vi "Configure Dialog.vi"(8 "error in (no error)":errorcluster, 11 "Get Auto Range Value [ARV] Msg.lvclass":refnum<class "Get Auto Range Value [ARV] Msg.lvclass">) -> (0 "error out":errorcluster, 2 "Ok?":bool, 3 "Get Auto Range Value [ARV] Msg.lvclass":refnum<class "Get Auto Range Value [ARV] Msg.lvclass">)   [LabVIEW 2015, in "CS++DMM.lvlib" / "Get Auto Range Value [ARV] Msg.lvclass"]
uses:
  Get Auto Range Value [ARV] Msg.lvclass
  Get Auto Range Value [ARV] Msg.lvclass/Get Auto Range Value [ARV] Msg.ctl
panel:
  in  "Execute?":bool
  in  "Cancel Button":bool
  in  "OK Button":bool
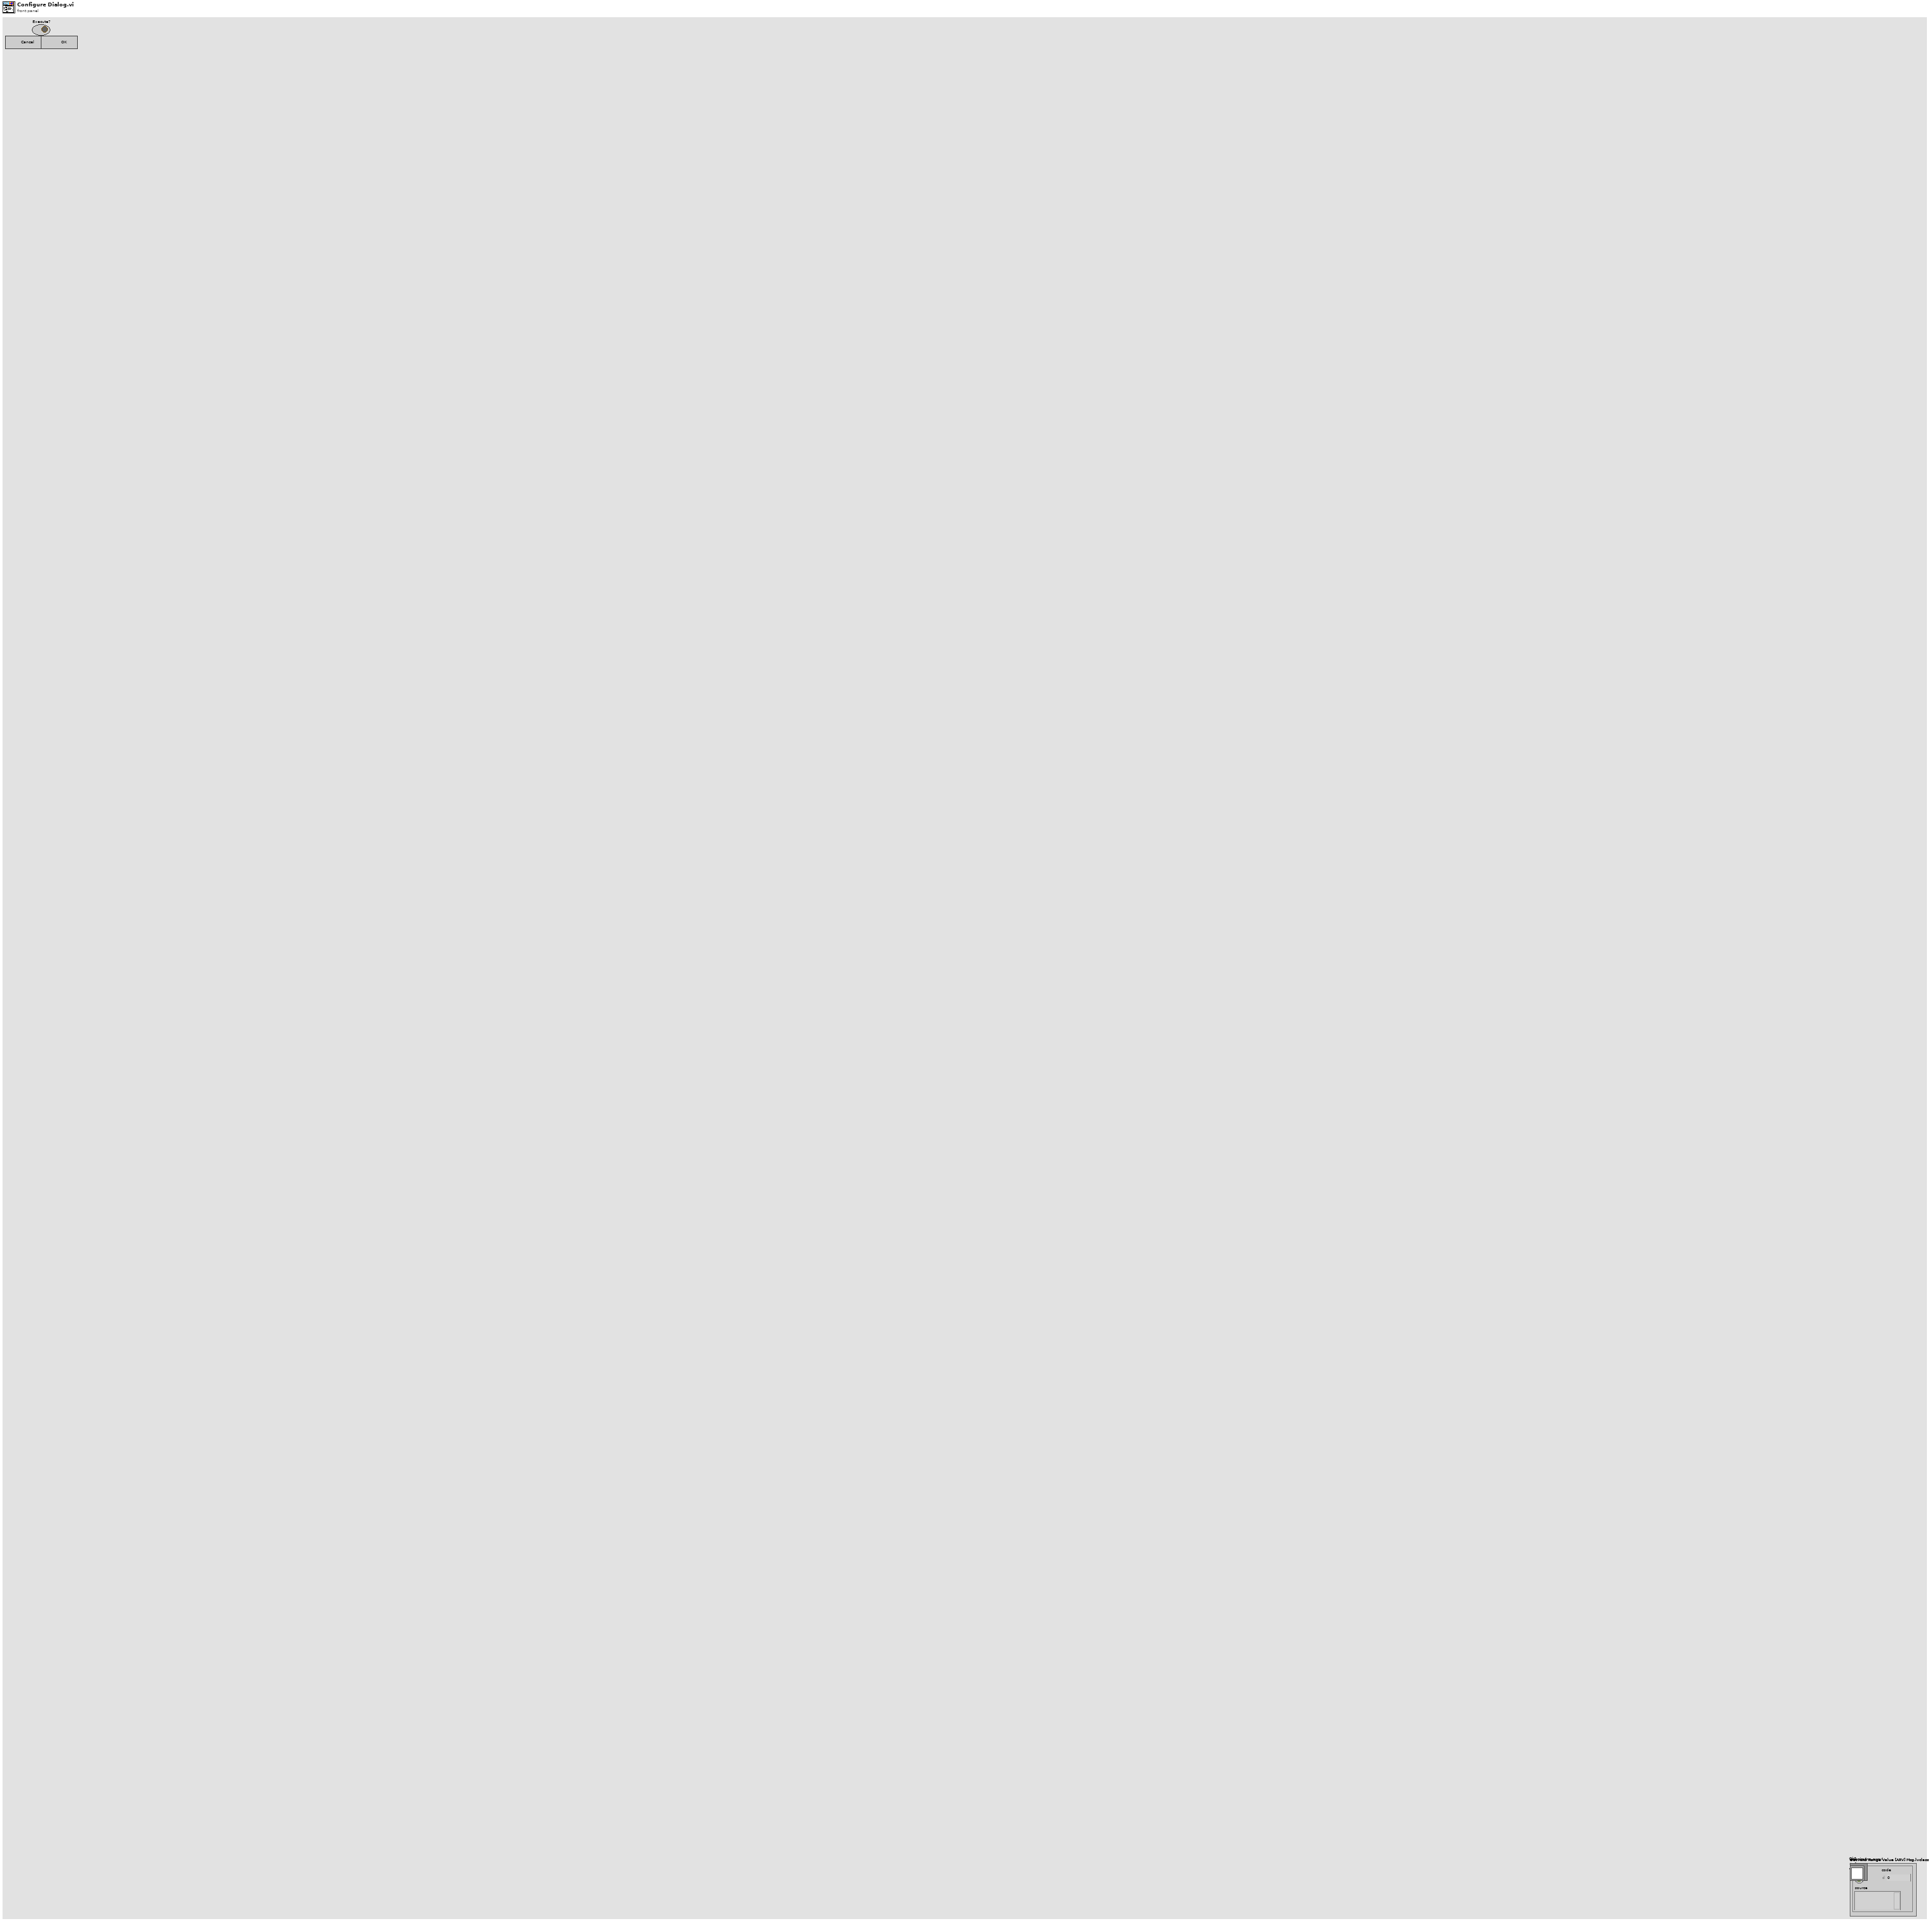
[diagram p1: front panel]
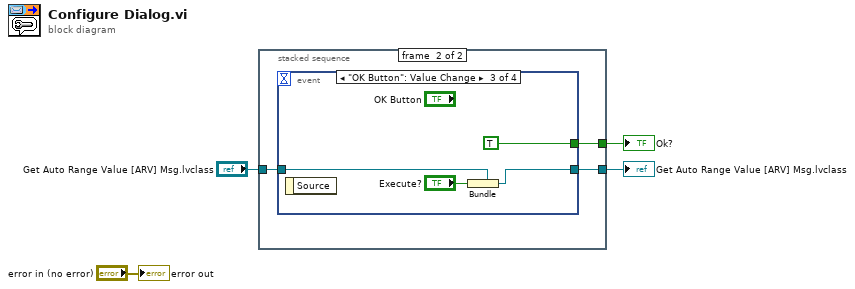
[diagram p0: block diagram]
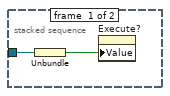
[diagram p2: hidden frame]
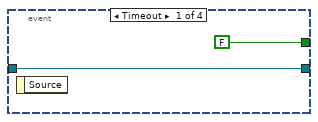
[diagram p3: hidden frame]
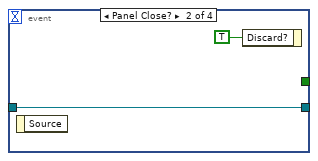
[diagram p4: hidden frame]
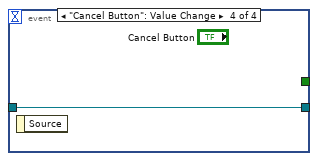
[diagram p5: hidden frame]
diagram:
  n1 = stacked-sequence {
    tunnel: [_ w9] -> w3
    tunnel: [_ w8] -> w2
    tunnel: "Get Auto Range Value [ARV] Msg.lvclass" -> [w6 w7]
    frame #0 {
      n2 = Unbundle ("Seq0Unbundler")(w6) -> (w5:bool)
      n3 = property on="Execute?" class="Bool (strict)"("Value"=w5) -> ()  [unwired: 2 in, 2 out]
    }
    frame #1 {
      n4 = event shown="[2] \"OK Button\": Value Change" {
        selector: _ -> [_ _ _ _]
        dyn-events: _ -> [_ _ _ _]
        timeout: _ -> [_ _ _ _]
        tunnel: [w10 w12 w15 w18] -> w8
        tunnel: w7 -> [w10 w12 w17 w18]
        tunnel: [FALSE _ TRUE _] -> w9
        event Timeout {
          n5 = event-data() -> ()  [unwired: 1 in, 1 out]
        }
        event Panel Close? {
          n6 = event-data() -> ()  [unwired: 1 in, 1 out]
          n7 = event-data ("Event Filter Node")("Discard?"=TRUE) -> ()  [unwired: 1 in, 1 out]
        }
        event "OK Button": Value Change {
          n8 = event-data() -> ()  [unwired: 1 in, 1 out]
          n9 = Bundle ("Main-Bundler")(cluster=w17, "Execute?") -> (w15:refnum<class "Get Auto Range Value [ARV] Msg.lvclass">)
        }
        event "Cancel Button": Value Change {
          n10 = event-data() -> ()  [unwired: 1 in, 1 out]
        }
      }
    }
  }
  "Ok?" <- w3
  "Get Auto Range Value [ARV] Msg.lvclass" <- w2
  "error out" <- "error in (no error)"
